vi "OverlayBitmapCenter.vi"(7 "GroupName":string, 8 "error in":errorcluster, 9 "Bitmap":u32[][](array[colorbox]), 10 "Center":T1, 11 "Image Reference In":T2) -> (0 "error out":errorcluster, 3 "Image Reference Out":T2)   [LabVIEW 2020, in "OpenLvVision_Overlays.lvlib"]
doc: "Overlays an bitmap on top of an image."
uses:
  OpenLvVision_Overlays.lvlib
  TypeDefs/PointI32.ctl
  <vilib>/OpenLvVision/OpenLvVision_Image/Management/TypeDef/OLV Image.ctl
  <vilib>/OpenLvVision/OpenLvVision_Image/Management/OLV Management.lvlib
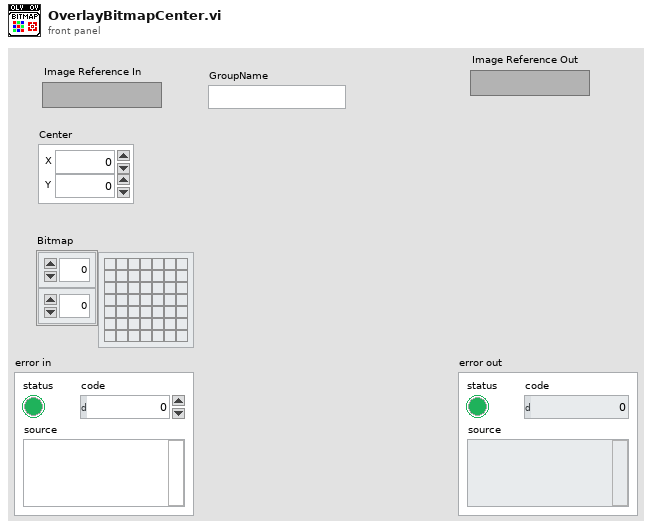
[diagram p1: front panel]
types:
  T1 = typedef "OpenLvVision_Overlays.lvlib/PointI32.ctl" = cluster{"X":i32, "Y":i32}
  T2 = typedef "OLV OpenLvVision_Image.lvlib/OLV Management.lvlib/OLV Image.ctl" = refnum<image>
  T3 = typedef "IMAQ Image.ctl" = refnum<image>
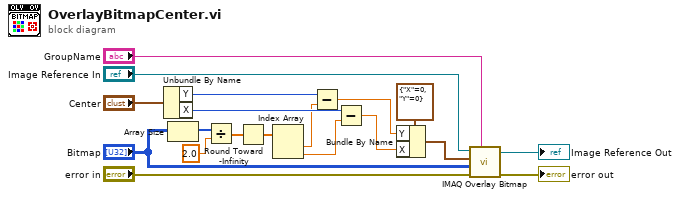
[diagram p0: block diagram]
diagram:
  n1 = Unbundle By Name("Center") -> ("Y"=w10:i32, "X"=w9:i32)
  n2 = Array Size(array="Bitmap") -> (size(s)=w13:i32[])
  n3 = Divide(x=w13, y=2.0) -> (x/y=w2:dbl[])
  n4 = Round Toward -Infinity(1:w2) -> (0:w1:dbl[])
  n5 = Index Array(array=w1) -> (element #1=w8:dbl, element #2=w7:dbl)  [unwired: 2 in]
  n6 = Subtract(x=w10, y=w8) -> (x-y=w5:dbl)
  n7 = Subtract(x=w9, y=w7) -> (x-y=w4:dbl)
  n8 = Bundle By Name(cluster=T1 {"X"=0, "Y"=0} ("Center"), "Y"=w5, "X"=w4) -> (w3:T1)
  n9 = call "IMAQ Overlay Bitmap"("Group"="GroupName", "error in (no error)"="error in", "Bitmap"="Bitmap", "Top Left Point"=w3, "Image"="Image Reference In") -> ("error out"=→"error out":errorcluster, "Image Out"=→"Image Reference Out":T3)  [unwired: 5 in]
